vi "GlobalWrite.vi"() -> ()   [LabVIEW 2013]
panel:
  in  "Writeout":dbl[](array[numeric])
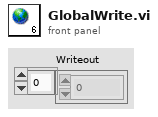
[diagram p1: front panel]
diagram:
